vi "data parsing(Voltage) from csv.vi"(11 "배열":string[](array[string])) -> (0 "Temp":u32[](array[numeric]), 1 "Battery":u32[](array[numeric]), 2 "No Filter Sensor":u32[][](array[numeric]), 3 "Time":string[](array[string]))   [LabVIEW 2015]
panel:
  out "No Filter Sensor 6":u32[](array[numeric])
  out "No Filter Sensor 5":u32[](array[numeric])
  out "No Filter Sensor 4":u32[](array[numeric])
  out "No Filter Sensor 3":u32[](array[numeric])
  out "No Filter Sensor 2":u32[](array[numeric])
  out "No Filter Sensor 1":u32[](array[numeric])
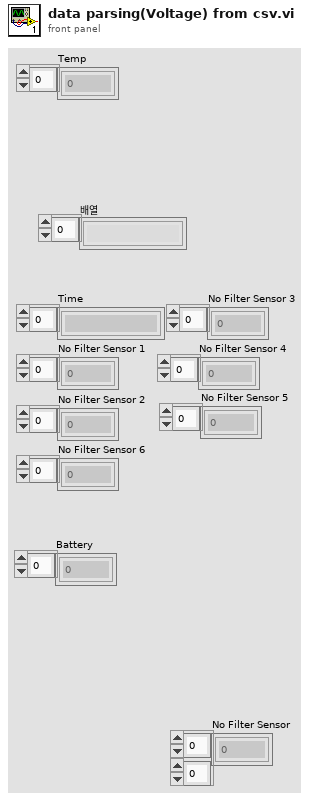
[diagram p1: front panel]
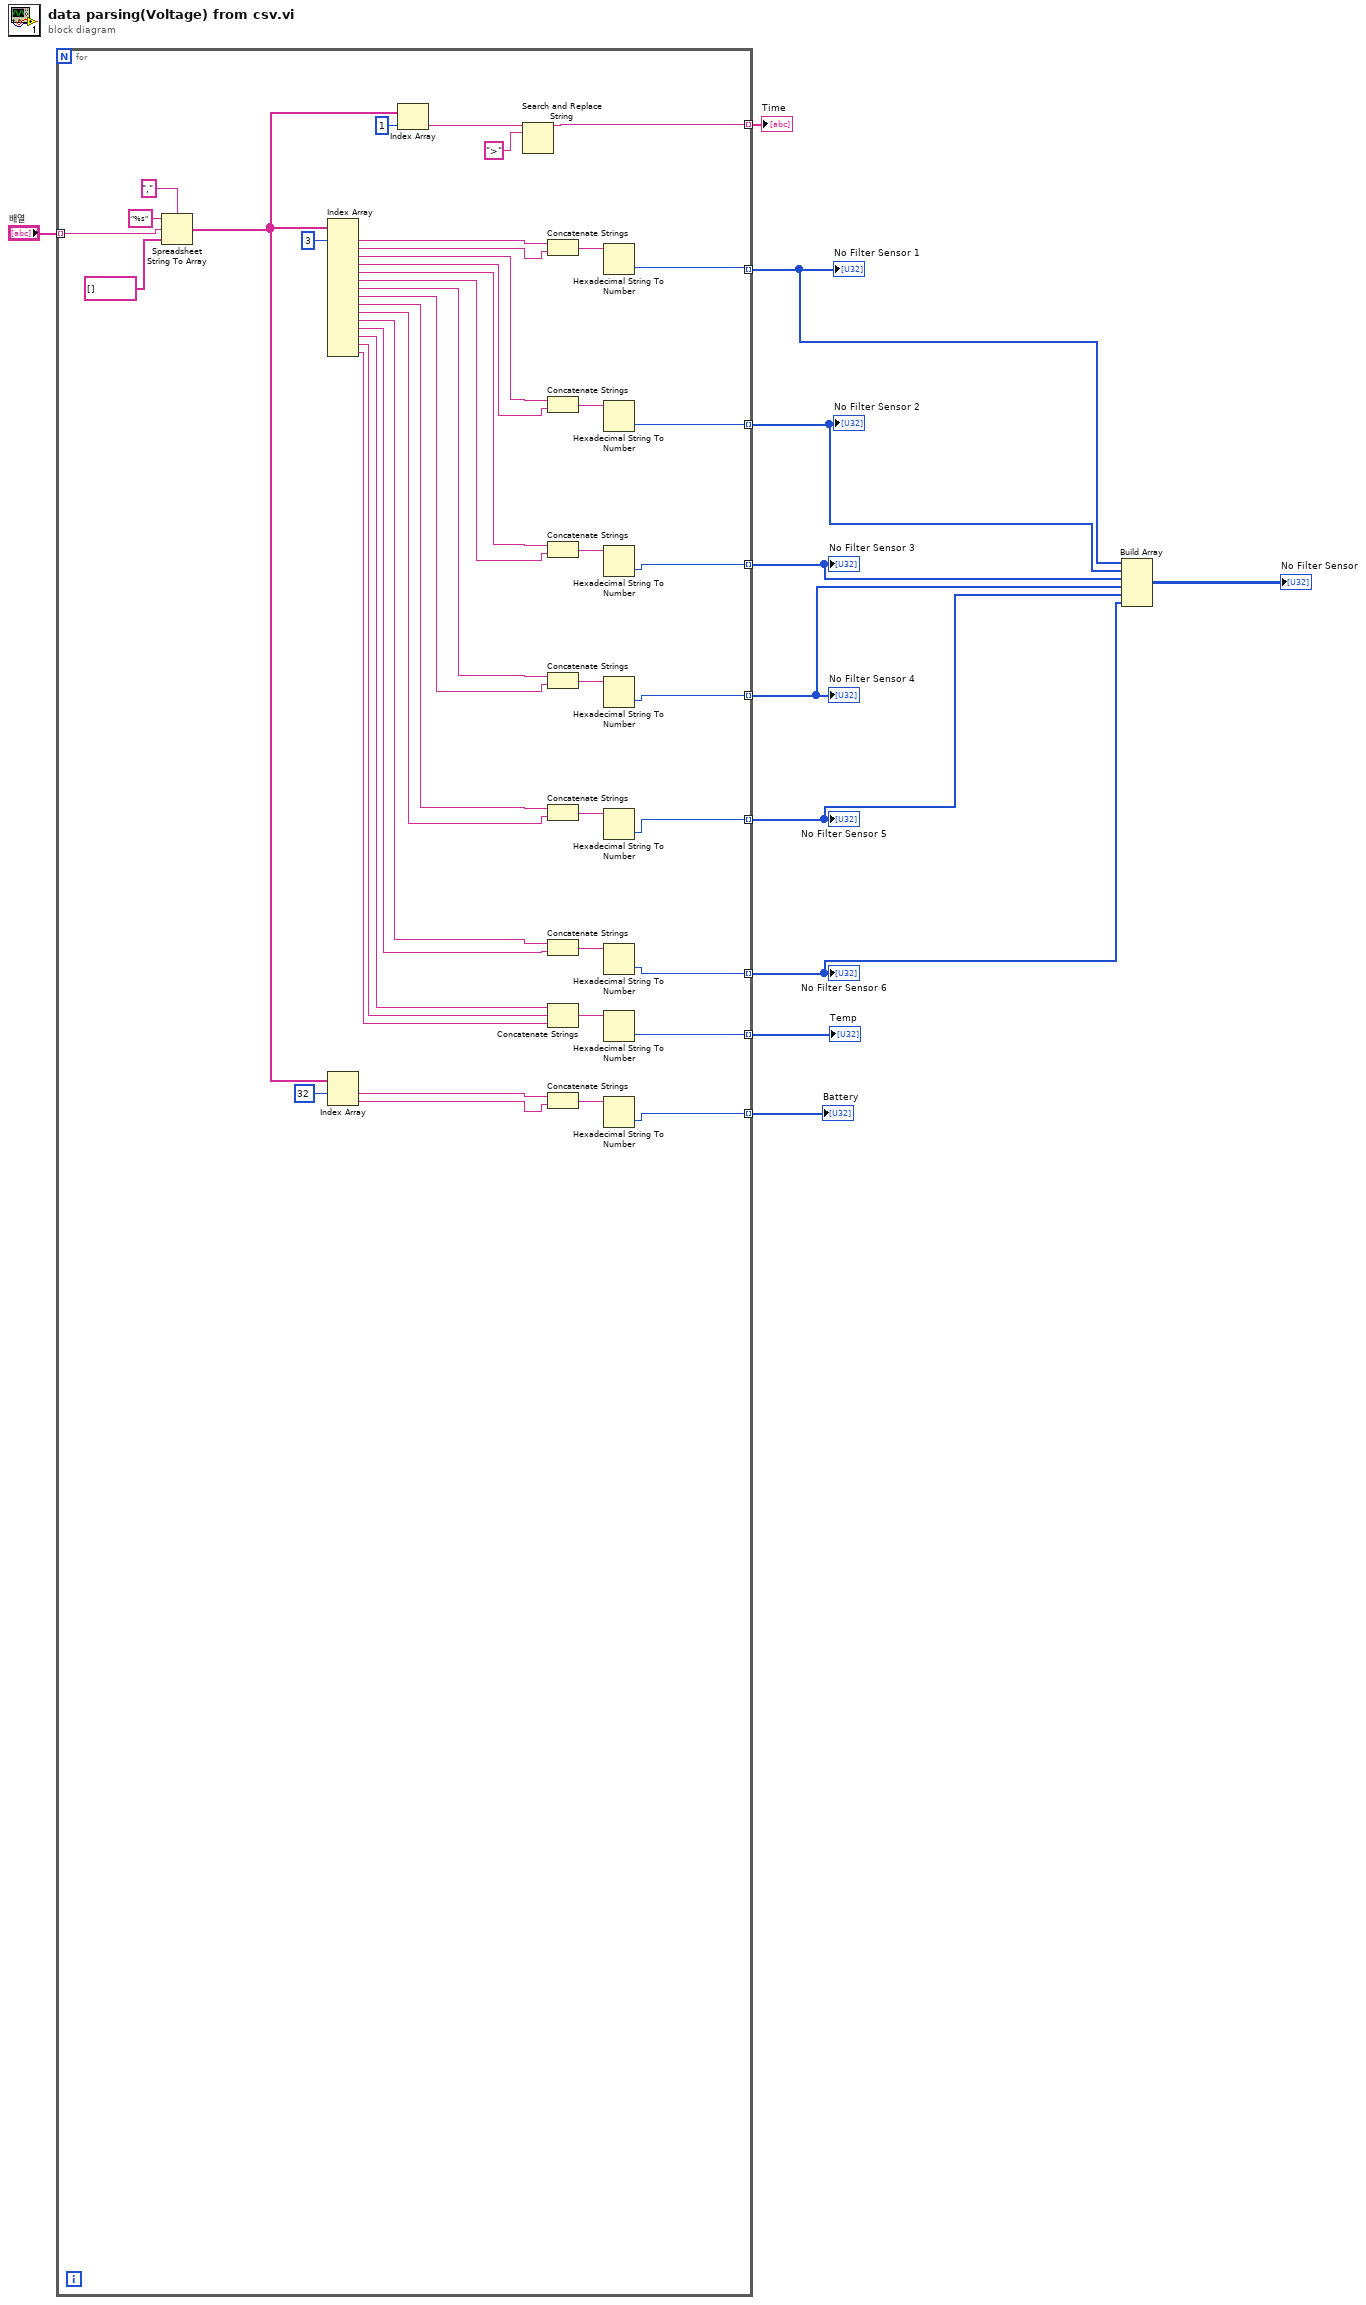
[diagram p0: block diagram]
diagram:
  n1 = for {
    tunnel: "배열" -> [w42] mode=indexing
    tunnel: [w31] -> w10 mode=indexing
    tunnel: [w23] -> w7 mode=indexing
    tunnel: [w22] -> w8 mode=indexing
    tunnel: [w21] -> w9 mode=indexing
    tunnel: [w20] -> w6 mode=indexing
    tunnel: [w19] -> w5 mode=indexing
    tunnel: [w18] -> w4 mode=indexing
    tunnel: [w17] -> w2 mode=indexing
    tunnel: [w12] -> w1 mode=indexing
    n2 = Spreadsheet String To Array(delimiter (Tab)="," ("구분 문자(탭)"), format string="%s" ("포맷 문자열"), spreadsheet string=w42, array type (2D Dbl)=string[] []) -> (array=w33:string[])
    n3 = Index Array(array=w33, index #1=3 ("비활성화된 인덱스 (열)")) -> (element #1=w55:string, element #2=w54:string, element #3=w53:string, element #4=w52:string, element #5=w51:string, element #6=w50:string, element #7=w49:string, element #8=w48:string, element #9=w47:string, element #10=w46:string, element #11=w38:string, element #12=w37:string, element #13=w15:string, element #14=w14:string, element #15=w13:string)  [unwired: 14 in]
    n4 = Index Array(array=w33, index #1=32 ("비활성화된 인덱스 (열)")) -> (element #1=w34:string, element #2=w35:string)  [unwired: 1 in]
    n5 = Index Array(array=w33, index=1 ("비활성화된 인덱스 (열)")) -> (element=w45:string)
    n6 = Search and Replace String(input string=w45, search string=">" ("검색 문자열")) -> (result string=w31:string)  [unwired: 6 in, 3 out]
    n7 = Concatenate Strings(w55, w54) -> (w30:string)
    n8 = Concatenate Strings(w53, w52) -> (w29:string)
    n9 = Concatenate Strings(w51, w50) -> (w28:string)
    n10 = Concatenate Strings(w49, w48) -> (w27:string)
    n11 = Concatenate Strings(w47, w46) -> (w26:string)
    n12 = Concatenate Strings(w38, w37) -> (w25:string)
    n13 = Concatenate Strings(w15, w14, w13) -> (w16:string)
    n14 = Concatenate Strings(w34, w35) -> (w24:string)
    n15 = Hexadecimal String To Number(string=w30) -> (number=w23:u32)  [unwired: 2 in, 1 out]
    n16 = Hexadecimal String To Number(string=w29) -> (number=w22:u32)  [unwired: 2 in, 1 out]
    n17 = Hexadecimal String To Number(string=w28) -> (number=w21:u32)  [unwired: 2 in, 1 out]
    n18 = Hexadecimal String To Number(string=w27) -> (number=w20:u32)  [unwired: 2 in, 1 out]
    n19 = Hexadecimal String To Number(string=w26) -> (number=w19:u32)  [unwired: 2 in, 1 out]
    n20 = Hexadecimal String To Number(string=w25) -> (number=w18:u32)  [unwired: 2 in, 1 out]
    n21 = Hexadecimal String To Number(string=w16) -> (number=w12:u32)  [unwired: 2 in, 1 out]
    n22 = Hexadecimal String To Number(string=w24) -> (number=w17:u32)  [unwired: 2 in, 1 out]
  }
  "Time" <- w10
  "No Filter Sensor 1" <- w7
  "No Filter Sensor 2" <- w8
  "No Filter Sensor 3" <- w9
  "No Filter Sensor 4" <- w6
  "No Filter Sensor 5" <- w5
  "No Filter Sensor 6" <- w4
  "Battery" <- w2
  "Temp" <- w1
  n23 = Build Array(w7, w8, w9, w6, w5, w4) -> (→"No Filter Sensor":u32[][])
